vi "Feed_Main.vi"(8 "error in (no error)":errorcluster, 11 "DevInfo":T1={"Hostname"="", "IPAddress"="", "MAC"="", "SerialNum"="", "Model"="", "Status"="", "FW"="", "OSDesc"="", "ImgTitle"="", "ImgDesc"="", "ImgVer"="", "ImgID"="", "IP Address Request Mode"=1, "SubnetMask"="", "Gateway"="", "DNSServer"=""} {"IP Address Request Mode" items=["Static"=1, "DHCP/Link-Local"=2, "Link-Local Only"=4, "DHCP Only"=8]}) -> (0 "error out":errorcluster)   [LabVIEW 2021]
uses:
  TypeDefs/DevInfo.ctl
  FeedSM_States.ctl
  TypeDefs/TargetAccess.ctl
  <vilib>/nisyscfg/Close (System).vi
  <vilib>/nisyscfg/nisyscfg.lvlib
panel:
  in  "Refresh Feeds":bool
  in  "Remove Feed":bool
  in  "Add Feed":bool
  in  "Feeds":i32(listbox)
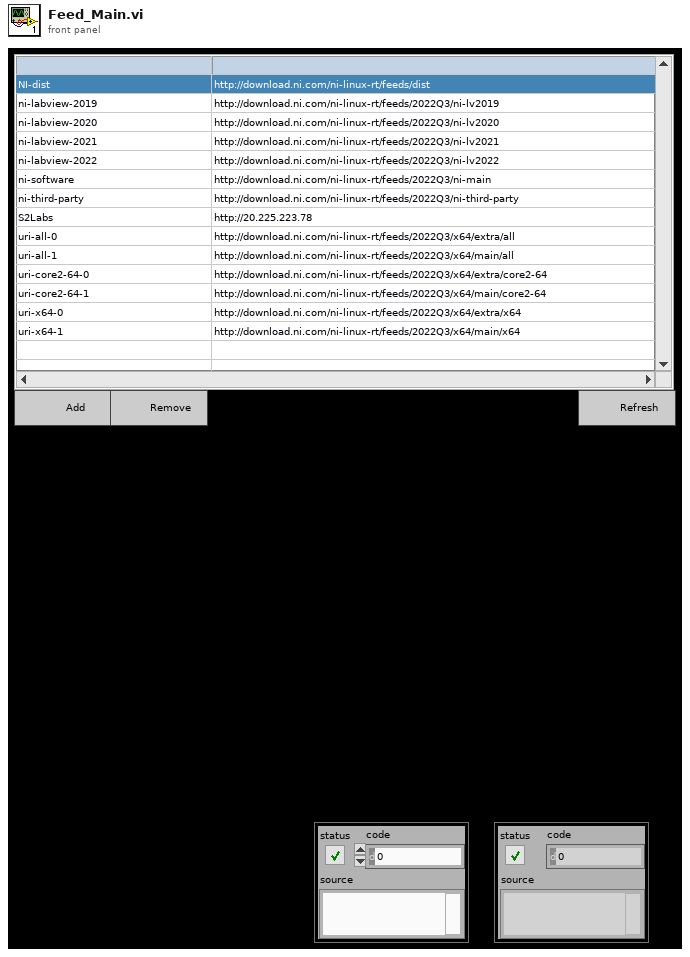
[diagram p1: front panel]
types:
  T1 = typedef "DevInfo.ctl" = cluster{"Hostname":string, "IPAddress":string, "MAC":string, "SerialNum":string, "Model":string, "Status":string, "FW":string, "OSDesc":string, "ImgTitle":string, "ImgDesc":string, "ImgVer":string, "ImgID":string, "IP Address Request Mode":i32, "SubnetMask":string, "Gateway":string, "DNSServer":string}
  T2 = typedef "FeedSM_States.ctl" = enum16{"Waiting", "Connect", "GetFeeds", "AddFeed", "RemoveFeed", "Exit"}
  T3 = typedef "TargetAccess.ctl" = enum16{"Read-Only", "Admin"}
  T4 = typedef "nisyscfg.lvlib/Software Feed.ctl" = cluster{"feed name":string, "uri":string, "enabled":bool, "trusted":bool}
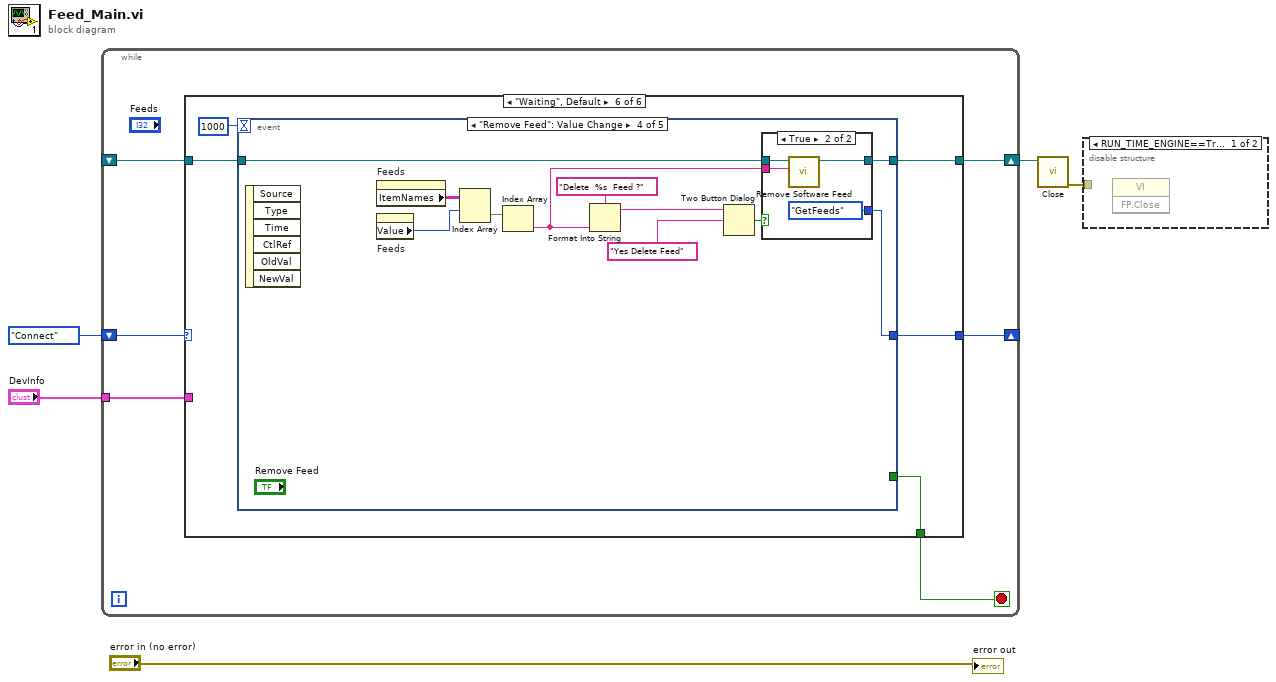
[diagram p0: block diagram]
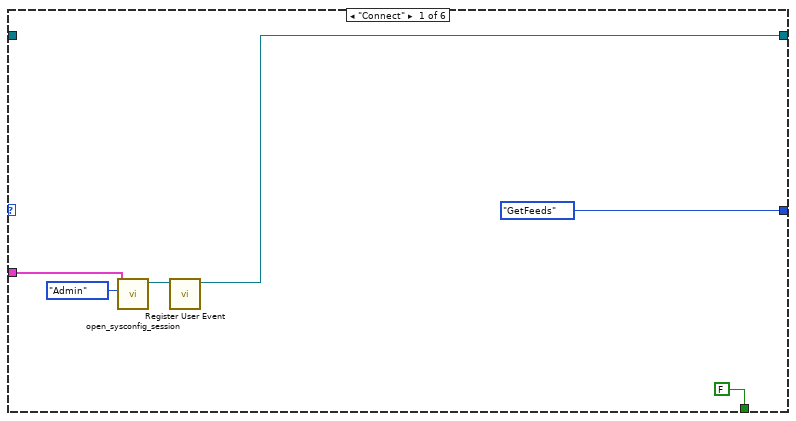
[diagram p3: hidden frame]
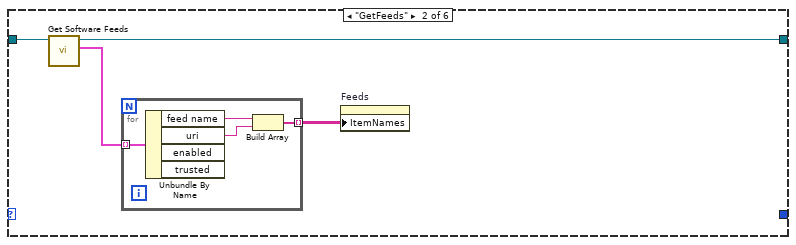
[diagram p4: hidden frame]
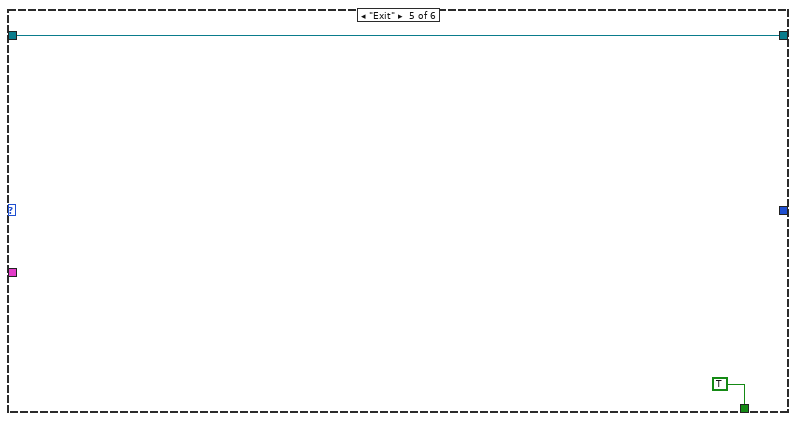
[diagram p7: hidden frame]
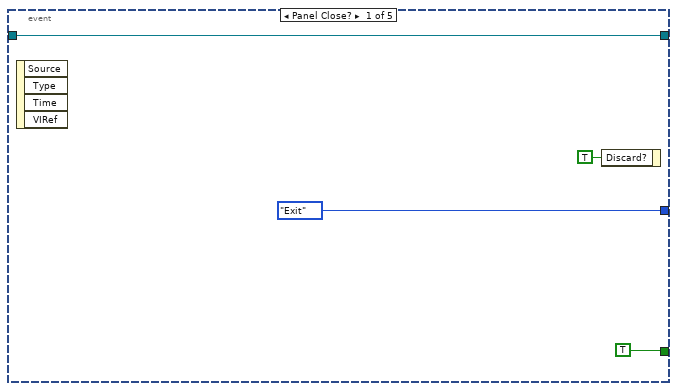
[diagram p8: hidden frame]
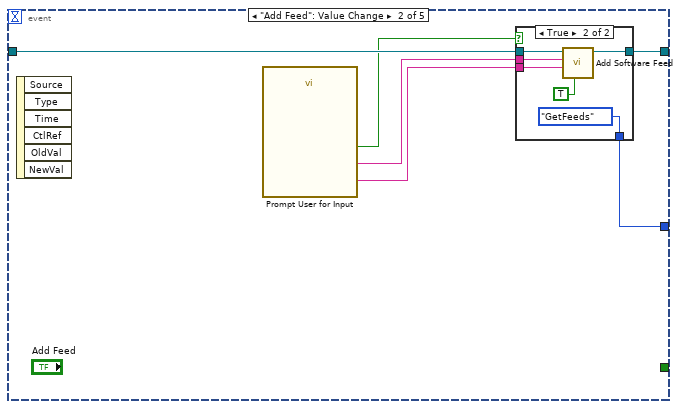
[diagram p9: hidden frame]
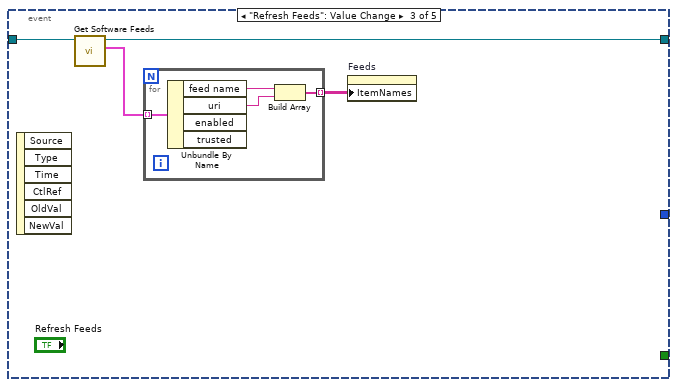
[diagram p11: hidden frame]
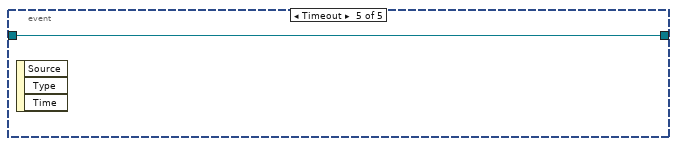
[diagram p13: hidden frame]
diagram:
  n1 = while {
    tunnel: "DevInfo" -> [w9]
    shift-right: [w6] -> _
    shift-left: FeedSM_States."Connect" -> [w11]
    shift-right: [w8] -> w2
    shift-left: _ -> [w7]
    stop <- w10 stop-if-true
    n2 = case shown="\"Waiting\", Default" w11 {
      tunnel: [FALSE _ _ _ TRUE w31] -> w10
      tunnel: w9 -> [w15 _ _ _ _ _]
      tunnel: [w14 w19 w26 w27 w29 w33] -> w8
      tunnel: w7 -> [_ w21 w26 w27 w29 w34]
      tunnel: [FeedSM_States."GetFeeds" _ _ _ _ w32] -> w6
      frame "Connect" {
        n3 = call "open_sysconfig_session.vi"("Target Access"=TargetAccess."Admin", "DevInfo"=w15) -> ("Session Out"=w17:refnum<k21>)  [unwired: 7 in, 2 out]
        n4 = call <vilib>:"Register User Event.vi"("Session in"=w17) -> ("Session out"=w14:refnum<k21>)  [unwired: 8 in, 2 out]
      }
      frame "GetFeeds" {
        n5 = call <vilib>:"Get Software Feeds.vi"("Session in"=w21) -> ("Software Feeds"=w20:T4[], "Session out"=w19:refnum<k21>)  [unwired: 8 in, 1 out]
        n6 = for {
          tunnel: w20 -> [w25] mode=indexing
          tunnel: [w22] -> w18 mode=indexing
          n7 = Unbundle By Name(w25) -> ("feed name"=w24:string, "uri"=w23:string)  [unwired: 2 out]
          n8 = Build Array(w24, w23) -> (w22:string[])
        }
        n9 = property on="Feeds" class="MCListbox (strict)"("ItemNames"=w18) -> ()  [unwired: 2 in, 2 out]
      }
      frame "AddFeed" {
      }
      frame "RemoveFeed" {
      }
      frame "Exit" {
      }
      frame "Waiting", Default {
        n10 = event shown="[3] \"Remove Feed\": Value Change" {
          selector: _ -> [_ _ _ _ _]
          dyn-events: _ -> [_ _ _ _ _]
          timeout: 1000 -> [_ _ _ _ _]
          tunnel: w34 -> [w38 w43 w54 w69 w76]
          tunnel: [w38 w44 w53 w70 w76] -> w33
          tunnel: [FeedSM_States."Exit" w39 _ w60 _] -> w32
          tunnel: [TRUE ("Discard?") _ _ _ _] -> w31
          event Panel Close? {
            n11 = event-data() -> ()  [unwired: 1 in, 4 out]
            n12 = event-data("Discard?"=TRUE) -> ()  [unwired: 1 in, 1 out]
          }
          event "Add Feed": Value Change {
            n13 = event-data() -> ()  [unwired: 1 in, 6 out]
            n14 = call "Prompt User for Input"() -> ("URI"=w41:string, "Feed Name"=w42:string, "OK"=w40:bool)  [unwired: 16 in, 1 out]
            n15 = case shown="True" w40 {
              tunnel: [w45 w50] -> w44
              tunnel: w43 -> [w45 w49]
              tunnel: w42 -> [_ w48]
              tunnel: w41 -> [_ w47]
              tunnel: [_ FeedSM_States."GetFeeds"] -> w39
              frame False {
              }
              frame True {
                n16 = call <vilib>:"Add Software Feed.vi"("Trusted (F)"=TRUE, "URI"=w47, "Feed Name"=w48, "Session in"=w49) -> ("Session out"=w50:refnum<k21>)  [unwired: 6 in, 1 out]
              }
            }
          }
          event "Refresh Feeds": Value Change {
            n17 = event-data() -> ()  [unwired: 1 in, 6 out]
            n18 = call <vilib>:"Get Software Feeds.vi"("Session in"=w54) -> ("Software Feeds"=w55:T4[], "Session out"=w53:refnum<k21>)  [unwired: 8 in, 1 out]
            n19 = for {
              tunnel: w55 -> [w59] mode=indexing
              tunnel: [w56] -> w52 mode=indexing
              n20 = Unbundle By Name(w59) -> ("feed name"=w58:string, "uri"=w57:string)  [unwired: 2 out]
              n21 = Build Array(w58, w57) -> (w56:string[])
            }
            n22 = property on="Feeds" class="MCListbox (strict)"("ItemNames"=w52) -> ()  [unwired: 2 in, 2 out]
          }
          event "Remove Feed": Value Change {
            n23 = event-data() -> ()  [unwired: 1 in, 6 out]
            n24 = property on="Feeds" class="MCListbox (strict)"() -> ("ItemNames"=w68:string[][])  [unwired: 2 in, 2 out]
            n25 = property on="Feeds" class="MCListbox (strict)"() -> ("Value"=w66:i32)  [unwired: 2 in, 2 out]
            n26 = Index Array(array=w68, index (row)=w66) -> (element=w67:string[])  [unwired: 1 in]
            n27 = Index Array(array=w67) -> (element=w61:string)  [unwired: 1 in]
            n28 = Format Into String(format string="Delete  %s  Feed ?", w61) -> (resulting string=w63:string)  [unwired: 2 in, 1 out]
            n29 = Two Button Dialog(message=w63, 2:"Yes Delete Feed" ("T button name (\"OK\")")) -> (T button?=w62:bool)  [unwired: 1 in]
            n30 = case shown="True" w62 {
              tunnel: [w71 w75] -> w70
              tunnel: w69 -> [w71 w74]
              tunnel: w61 -> [_ w73]
              tunnel: [_ FeedSM_States."GetFeeds"] -> w60
              frame False {
              }
              frame True {
                n31 = call <vilib>:"Remove Software Feed.vi"("Feed Name"=w73, "Session in"=w74) -> ("Session out"=w75:refnum<k21>)  [unwired: 8 in, 1 out]
              }
            }
          }
          event Timeout {
            n32 = event-data() -> ()  [unwired: 1 in, 3 out]
          }
        }
      }
    }
  }
  n33 = call-poly <vilib>:"Close.vi"("Session in"=w2) -> ("error out"=w1:errorcluster)  [unwired: 10 in]
  n34 = disable-structure shown="RUN_TIME_ENGINE==True" {
    disable-tunnel: w1 -> [_ _]
    frame condition #0 {
      n35 = invoke class="VI" method="FP.Close"() -> ()  [unwired: 3 in, 3 out]
    }
    frame condition #1 (active) {
    }
  }
  "error out" <- "error in (no error)"
